vi "DecodeTimeStamp.vi"(11 "String in":string) -> (2 "Remaining String":string, 3 "time stamp":timestamp)   [LabVIEW 2024]
uses:
  <vilib>/Utility/miscctls.llb/LVDateTimeRec.ctl
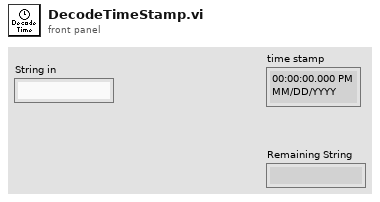
[diagram p1: front panel]
types:
  T1 = typedef "LVDateTimeRec.ctl" = cluster{"fractional second":dbl, "second":i32, "minute":i32, "hour":i32, "day of month":i32, "month":i32, "year":i32, "day of week":i32, "day of year":i32, "DST":i32}
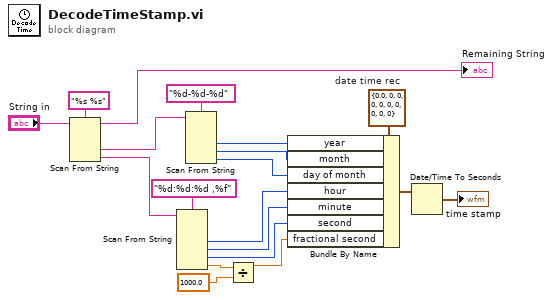
[diagram p0: block diagram]
diagram:
  w19 = T1 {"fractional second"=0.0, "second"=0, "minute"=0, "hour"=0, "day of month"=0, "month"=0, "year"=0, "day of week"=0, "day of year"=0, "DST"=0}  # date time rec
  n1 = Scan From String(format string="%s %s", input string="String in") -> (remaining string=→"Remaining String":string, output 1=w3:string, output 2=w10:string)  [unwired: 4 in, 2 out]
  n2 = Scan From String(format string="%d:%d:%d ,%f", input string=w10) -> (output 1=w13:i32, output 2=w12:i32, output 3=w14:i32, output 4=w15:dbl)  [unwired: 6 in, 3 out]
  n3 = Scan From String(format string="%d-%d-%d", input string=w3) -> (output 1=w5:i32, output 2=w6:i32, output 3=w7:i32)  [unwired: 5 in, 3 out]
  n4 = Divide(x=w15, y=1000.0 ("x")) -> (x/y=w16:dbl)
  n5 = Bundle By Name(cluster=w19, "year"=w5, "month"=w6, "day of month"=w7, "hour"=w13, "minute"=w12, "second"=w14, "fractional second"=w16) -> (w9:T1)
  n6 = Date/Time To Seconds(2:w9) -> (0:→"time stamp":timestamp)  [unwired: 1 in]
